vi "Save to file.vi"(8 "error in (no error)":errorcluster, 10 "Report Directory":path, 11 "Report Generator In":refnum<class "Report Generator.lvclass">) -> (0 "error out":errorcluster, 3 "Report Generator Out":refnum<class "Report Generator.lvclass">)   [LabVIEW 2020, in "Report Generator.lvclass"]
uses:
  Report Generator.lvclass
  C:/Git/astemes-lunit/source/Application Framework/Process Classes/Process/Process.lvclass
  Application Framework/Process Classes/Process/Process.lvclass/Process.ctl
  Application Framework/Process Classes/Process/Process.lvclass
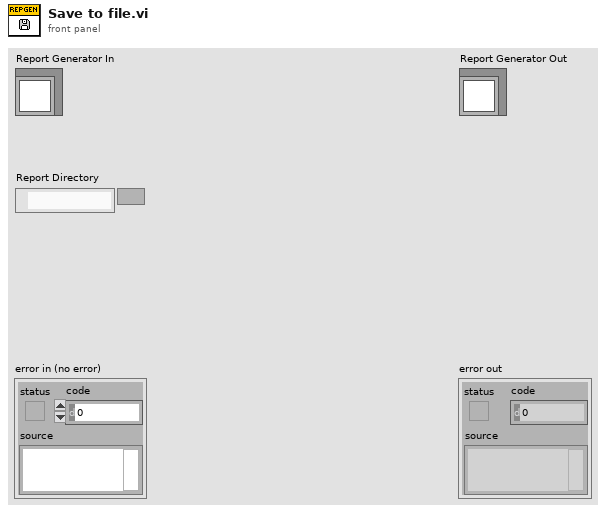
[diagram p1: front panel]
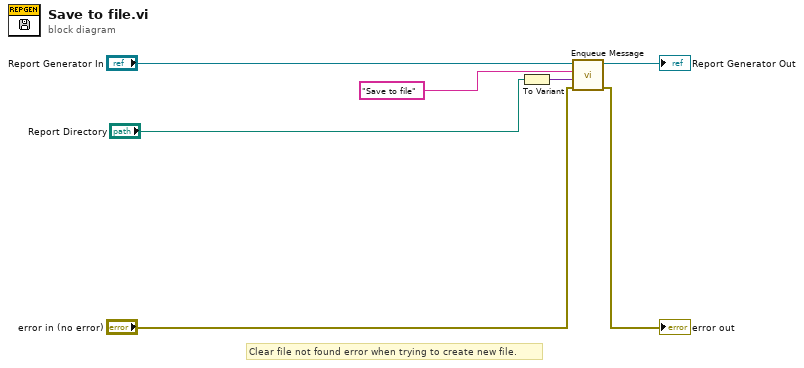
[diagram p0: block diagram]
diagram:
  # "Clear file not found error when trying to create new file."
  n1 = To Variant(anything="Report Directory") -> (Variant=w3:variant)
  n2 = call "Enqueue Message.vi"("error in (no error)"="error in (no error)", "Message Data"=w3, "Message"="Save to file", "Process In"="Report Generator In") -> ("error out"=→"error out":errorcluster, "Process Out"=→"Report Generator Out":refnum<class "Report Generator.lvclass">)  [unwired: 6 in]
